vi "ReadWrite.Lookup.vi"(8 "error in (no error)":errorcluster, 10 "Name":string, 11 "Data Access API in":refnum<class "Data Access Engine.lvclass">) -> (0 "error out":errorcluster, 2 "Ref":refnum<data-value>, 3 "Data Access API out":refnum<class "Data Access Engine.lvclass">)   [LabVIEW 2015, in "Data Access Engine.lvlib" / "Data Access Engine.lvclass"]
uses:
  Data Access Engine.lvclass
  Data/ReadWrite/ReadWrite.lvclass
  Data Access Engine.lvclass/Data Access Engine.ctl
  Types/VS Channel Group Type.ctl
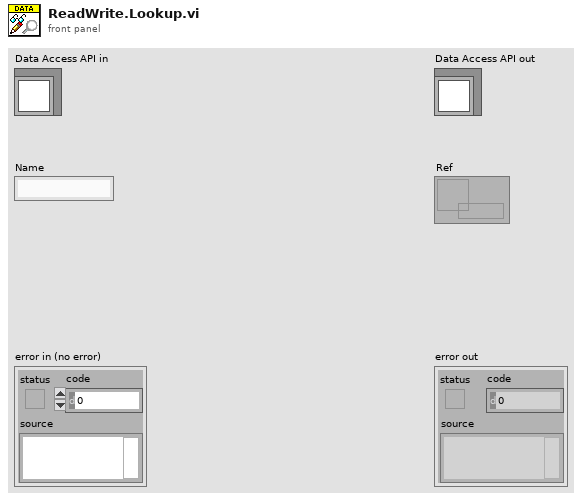
[diagram p1: front panel]
types:
  T1 = typedef "Data Access Engine.lvlib/Data Access Engine.lvclass/VS Channel Group Type.ctl" = enum16{"Output/Write", "Input/Read", "Input/ReadWrite"}
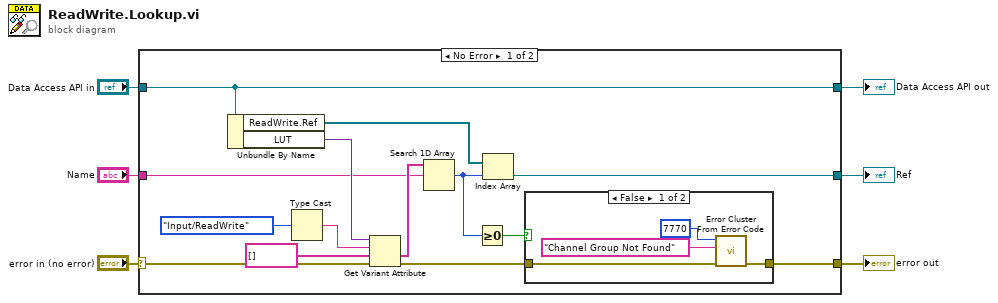
[diagram p0: block diagram]
diagram:
  n1 = case shown="No Error" "error in (no error)" {
    selector: "error in (no error)" -> [w15 w27]
    tunnel: [w7 w27] -> w5
    tunnel: [w20 w26] -> w3
    tunnel: "Data Access API in" -> [w20 w26]
    tunnel: "Name" -> [w13 _]
    tunnel: [w11 _] -> w1
    frame No Error {
      n2 = Unbundle By Name(w20) -> ("ReadWrite.Ref"=w12:refnum<data-value>[], "LUT"=w19:variant)
      n3 = Type Cast(x=VS_Channel_Group_Type."Input/ReadWrite" ("Type")) -> (*(type *) &x=w17:string)  [unwired: 1 in]
      n4 = Get Variant Attribute(Variant=w19, name=w17, default value (empty Variant)=string[] [], error in=w15) -> (value=w14:string[], error out=w9:errorcluster)  [unwired: 2 out]
      n5 = Search 1D Array(1D array=w14, element=w13) -> (index of element=w10:i32)  [unwired: 1 in]
      n6 = Greater Or Equal To 0?(x=w10) -> (x >= 0?=w8:bool)
      n7 = Index Array(array=w12, index=w10) -> (element=w11:refnum<data-value>)
      n8 = case shown="False" w8 {
        tunnel: w9 -> [w24 w25]
        tunnel: [w23 w25] -> w7
        frame False {
          n9 = call <vilib>:"Error Cluster From Error Code.vi"("error in (no error)"=w24, "error message (\"\")"="Channel Group Not Found" ("error message (\"\")"), "error code (0)"=7770) -> ("error out"=w23:errorcluster)  [unwired: 6 in]
        }
        frame True {
        }
      }
    }
    frame Error {
    }
  }
  "error out" <- w5
  "Data Access API out" <- w3
  "Ref" <- w1
